vi "Configure Digital Input Attenuation.vi"(8 "error in (no error)":errorcluster, 9 "Input Attenuation (0.00000000E+0 dB)":dbl format="%.8e", 10 "Auto Input Attenuation (T: Enable)":bool=TRUE, 11 "VISA resource name":refnum<visa-resource-name>) -> (0 "error out":errorcluster, 3 "VISA resource name out":refnum<visa-resource-name>)   [LabVIEW 2018, in "Agilent PSG MXG Series.lvlib"]
doc: "Configures the digital signal input attenuation.\n\n<b>Note:</b>\nIt is applicable for N5172B/82B with <b>Option 004</b> only."
uses:
  Agilent PSG MXG Series.lvlib
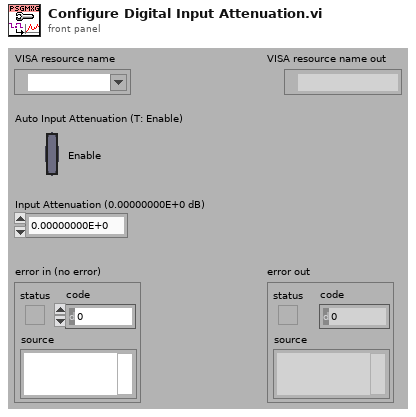
[diagram p1: front panel]
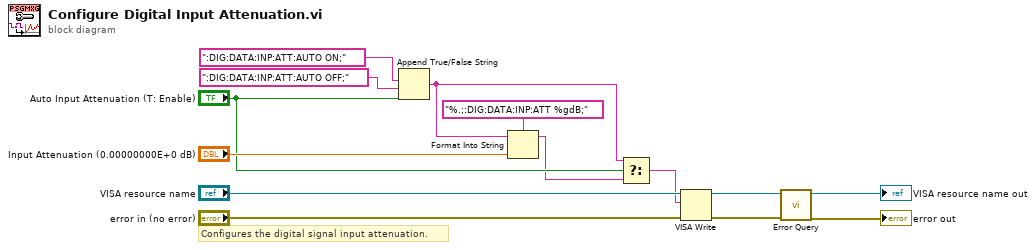
[diagram p0: block diagram]
diagram:
  # "Configures the digital signal input attenuation."
  n1 = Append True/False String(1:"Auto Input Attenuation (T: Enable)", 2:":DIG:DATA:INP:ATT:AUTO OFF;", 3:":DIG:DATA:INP:ATT:AUTO ON;") -> (0:w3:string)  [unwired: 1 in]
  n2 = Format Into String(format string="%.;:DIG:DATA:INP:ATT %gdB;", initial string=w3, "Input Attenuation (0.00000000E+0 dB)") -> (resulting string=w2:string)  [unwired: 1 in, 1 out]
  n3 = Select(t=w3, s="Auto Input Attenuation (T: Enable)", f=w2) -> (s? t:f=w1:string)
  n4 = VISA Write(VISA resource name="VISA resource name", write buffer=w1, error in (no error)="error in (no error)") -> (VISA resource name out=w8:refnum<visa-resource-name>, error out=w7:errorcluster)  [unwired: 1 out]
  n5 = call "Error Query.vi"("error in (no error)"=w7, "VISA resource name"=w8) -> ("error out"=→"error out":errorcluster, "VISA resource name out"=→"VISA resource name out":refnum<visa-resource-name>)  [unwired: 6 in, 2 out]
